vi "harp_connection_open.vi"(0 "Port:":refnum<visa-resource-name>="COMx", 1 "device's firmware name":string, 2 "launch dialog":bool, 3 ".X settings":T2={"fw .hex file path"=path "Fir", "updater path"=path "Fir"}, 7 "Expected device ID":u16=1024, 11 "MinimumVersions":T3={"hwVerMajor"=0, "fwVerMajor"=0, "harpVerMajor"=0, "assVer"=0, "hwVerMinor"=0, "fwVerMinor"=0, "harpVerMinor"=10}, 12 "get lists only":bool, 13 "baud rate":u32(ring)=1000000 items=["250Kbit/s"=250000, "500kbit/s"=500000, "1Mbit/s"=1000000, "2Mbit/s"=2000000, "4Mbit/s"=4000000]) -> (4 "port out":refnum<visa-resource-name>, 6 "Devices Name List":string[](array[string])=["Not defined", "Poke", "Multi Pwm Generator", "Wear", "12 Volts Drive", "LED Controller", "Synchronizer", "Simple Analog Generator", "Archimedes", "Clock Synchronizer", "Camera Controller", "Behavior"], 8 "cancel (T)":bool caption="Boolean", 10 "Devices WhoAmI List":u16[](array[numeric])=[0, 1024, 1040, 1056, 1072, 1088, 1104, 1121, 1136, 1152, 1168, 1216], 14 "Devices X. settings":T1(array[cluster])=[{"reg. address"=0, "address content (en)"=0, "address content (dis)"=0, "Has .X"=FALSE}, {"reg. address"=0, "address content (en)"=0, "address content (dis)"=0, "Has .X"=FALSE}, {"reg. address"=0, "address content (en)"=0, "address content (dis)"=0, "Has .X"=FALSE}, {"reg. address"=0, "address content (en)"=0, "address content (dis)"=0, "Has .X"=FALSE}, {"reg. address"=0, "address content (en)"=0, "address content (dis)"=0, "Has .X"=FALSE}, {"reg. address"=0, "address content (en)"=0, "address content (dis)"=0, "Has .X"=FALSE}, {"reg. address"=0, "address content (en)"=0, "address content (dis)"=0, "Has .X"=FALSE}, {"reg. address"=0, "address content (en)"=0, "address content (dis)"=0, "Has .X"=FALSE}, {"reg. address"=0, "address content (en)"=0, "address content (dis)"=0, "Has .X"=FALSE}, {"reg. address"=0, "address content (en)"=0, "address content (dis)"=0, "Has .X"=FALSE}, {"reg. address"=0, "address content (en)"=0, "address content (dis)"=0, "Has .X"=FALSE}, {"reg. address"=0, "address content (en)"=0, "address content (dis)"=0, "Has .X"=FALSE}, {"reg. address"=0, "address content (en)"=0, "address content (dis)"=0, "Has .X"=FALSE}, {"reg. address"=0, "address content (en)"=0, "address content (dis)"=0, "Has .X"=FALSE}, {"reg. address"=0, "address content (en)"=0, "address content (dis)"=0, "Has .X"=FALSE}, {"reg. address"=82, "address content (en)"=1, "address content (dis)"=0, "Has .X"=TRUE}, {"reg. address"=0, "address content (en)"=0, "address content (dis)"=0, "Has .X"=FALSE}], 15 "error out":errorcluster)   [LabVIEW 2010]
uses:
  <vilib>/Instr/_visa.llb/VISA Flush IO Buffer Mask.ctl
  <vilib>/Instr/_visa.llb/VISA Configure Serial Port (Instr).vi
panel:
  in  "cancel":bool caption="Boolean"
  in  "connect":bool caption="Boolean"
  # "Choose the device COM port."
  # "COM port:"
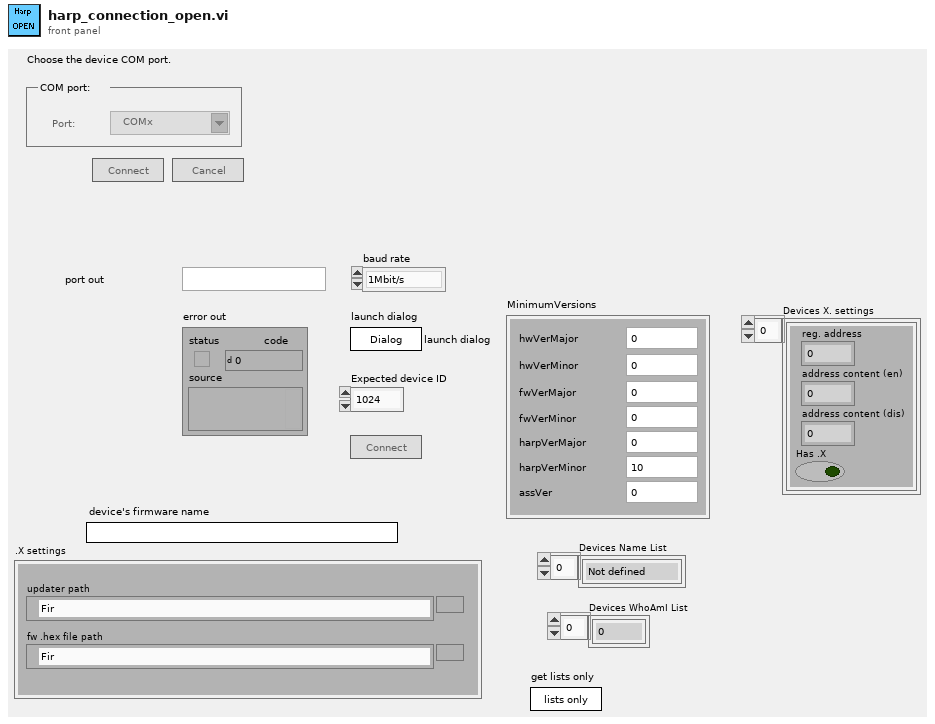
[diagram p1: front panel]
types:
  T1 = cluster{"reg. address":u8, "address content (en)":u8, "address content (dis)":u8, "Has .X":bool}[]
  T2 = cluster{"fw .hex file path":path, "updater path":path}
  T3 = cluster{"hwVerMajor":u8, "fwVerMajor":u8, "harpVerMajor":u8, "assVer":u8, "hwVerMinor":u8, "fwVerMinor":u8, "harpVerMinor":u8}
  T4 = cluster{"reg. address":u8, "address content (en)":u8, "address content (dis)":u8, "fw .hex file path":path, "updater path":path}
  T5 = enum8{"Enabled", "Disabled", "Disabled and Grayed Out"}
  T6 = typedef "VISA Flush IO Buffer Mask.ctl" = u16
  T7 = cluster{"reg. address":u8, "address content (en)":u8, "address content (dis)":u8, "Has .X":bool}
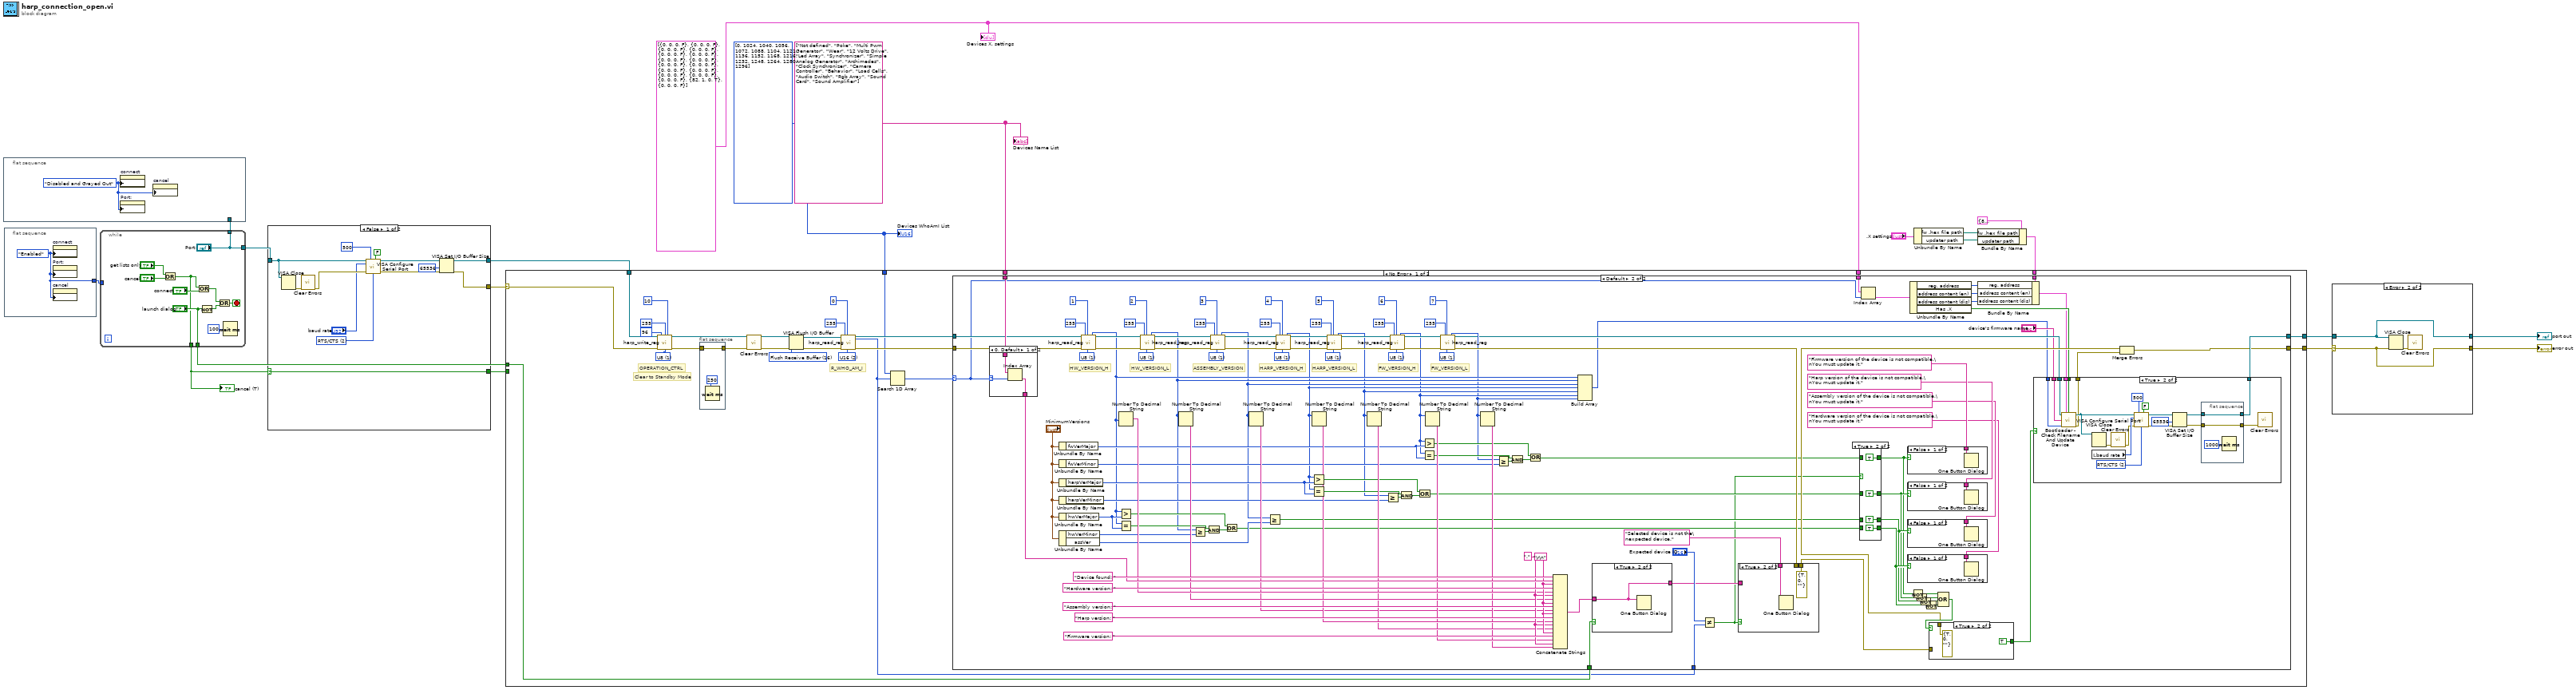
[diagram p0: block diagram]
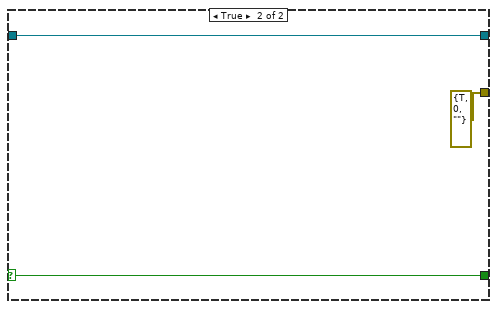
[diagram p3: hidden frame]
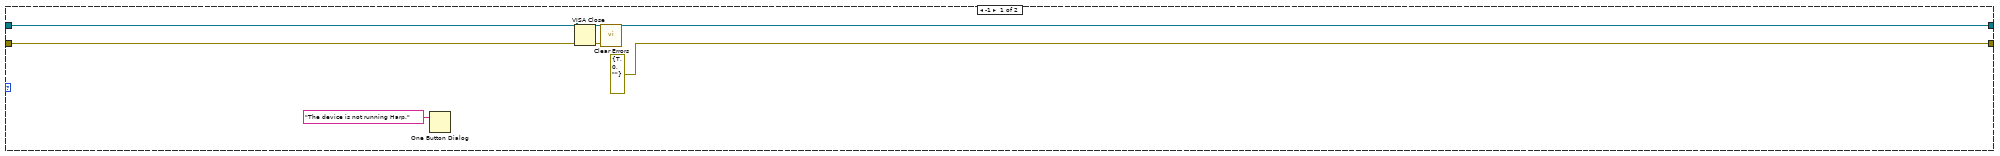
[diagram p4: hidden frame]
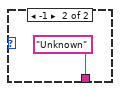
[diagram p5: hidden frame]
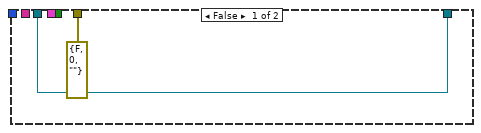
[diagram p6: hidden frame]
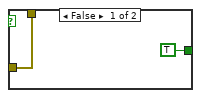
[diagram p8: hidden frame]
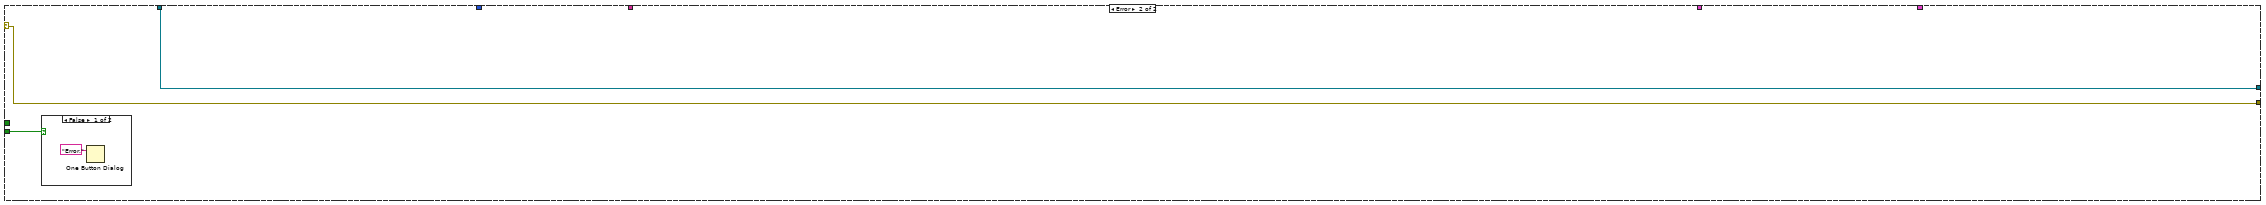
[diagram p15: hidden frame]
diagram:
  w6 = T1 [{"reg. address"=0, "address content (en)"=0, "address content (dis)"=0, "Has .X"=FALSE}, {"reg. address"=0, "address content (en)"=0, "address content (dis)"=0, "Has .X"=FALSE}, {"reg. address"=0, "address content (en)"=0, "address content (dis)"=0, "Has .X"=FALSE}, {"reg. address"=0, "address content (en)"=0, "address content (dis)"=0, "Has .X"=FALSE}, {"reg. address"=0, "address content (en)"=0, "address content (dis)"=0, "Has .X"=FALSE}, {"reg. address"=0, "address content (en)"=0, "address content (dis)"=0, "Has .X"=FALSE}, {"reg. address"=0, "address content (en)"=0, "address content (dis)"=0, "Has .X"=FALSE}, {"reg. address"=0, "address content (en)"=0, "address content (dis)"=0, "Has .X"=FALSE}, {"reg. address"=0, "address content (en)"=0, "address content (dis)"=0, "Has .X"=FALSE}, {"reg. address"=0, "address content (en)"=0, "address content (dis)"=0, "Has .X"=FALSE}, {"reg. address"=0, "address content (en)"=0, "address content (dis)"=0, "Has .X"=FALSE}, {"reg. address"=0, "address content (en)"=0, "address content (dis)"=0, "Has .X"=FALSE}, {"reg. address"=0, "address content (en)"=0, "address content (dis)"=0, "Has .X"=FALSE}, {"reg. address"=0, "address content (en)"=0, "address content (dis)"=0, "Has .X"=FALSE}, {"reg. address"=0, "address content (en)"=0, "address content (dis)"=0, "Has .X"=FALSE}, {"reg. address"=82, "address content (en)"=1, "address content (dis)"=0, "Has .X"=TRUE}, {"reg. address"=0, "address content (en)"=0, "address content (dis)"=0, "Has .X"=FALSE}] ("Array")
  w18 = string[] ["Not defined", "Poke", "Multi Pwm Generator", "Wear", "12 Volts Drive", "Led Array", "Synchronizer", "Simple Analog Generator", "Archimedes", "Clock Synchronizer", "Camera Controller", "Behavior", "Load Cells", "Audio Switch", "Rgb Array", "Sound Card", "Sound Amplifier"]
  w19 = u16[] [0, 1024, 1040, 1056, 1072, 1088, 1104, 1121, 1136, 1152, 1168, 1216, 1232, 1248, 1264, 1280, 1296]
  n1 = flat-sequence {
    tunnel: w13 -> [_]
    frame #0 {
      w21 = T5."Disabled and Grayed Out" ("Disabled")
      n2 = property on="connect" class="Bool"("DisabledEnum"=w21) -> ()  [unwired: 2 in, 2 out]
      n3 = property on="Port:" class="VISAName"("DisabledEnum"=w21) -> ()  [unwired: 2 in, 2 out]
      n4 = property on="cancel" class="Bool"("DisabledEnum"=w21) -> ()  [unwired: 2 in, 2 out]
    }
  }
  n5 = flat-sequence {
    tunnel: [w22] -> w14
    frame #0 {
      w22 = T5."Enabled" ("Disabled")
      n6 = property on="connect" class="Bool"("DisabledEnum"=w22) -> ()  [unwired: 2 in, 2 out]
      n7 = property on="Port:" class="VISAName"("DisabledEnum"=w22) -> ()  [unwired: 2 in, 2 out]
      n8 = property on="cancel" class="Bool"("DisabledEnum"=w22) -> ()  [unwired: 2 in, 2 out]
    }
  }
  n9 = while {
    tunnel: ["Port:"] -> w17
    tunnel: ["launch dialog"] -> w20
    tunnel: w14 -> [_]
    tunnel: ["Port:"] -> w13
    tunnel: [w24] -> w12
    stop <- w31 stop-if-true
    n10 = Or(x="get lists only", y="cancel") -> (x .or. y?=w24:bool)
    n11 = Or(x=w24, y="connect") -> (x .or. y?=w26:bool)
    n12 = Not(x="launch dialog") -> (.not. x?=w30:bool)
    n13 = Or(x=w26, y=w30) -> (x .or. y?=w31:bool)
    n14 = Wait (ms)(milliseconds to wait=u32 100) -> ()  [unwired: 1 out]
  }
  "cancel (T)" <- w12
  n15 = case shown="False" w12 {
    selector: w12 -> [w33 w46]
    tunnel: w17 -> [w39 w48]
    tunnel: [w36 errorcluster {"status"=TRUE, "code"=0, "source"=""} ("error out")] -> w16
    tunnel: [w35 w48] -> w15
    tunnel: [w33 w46] -> w11
    frame False {
      w41 = u16 2 items=["None", "XON/XOFF", "RTS/CTS", "XON/XOFF & RTS/CTS", "DTR/DSR", "XON/XOFF & DTR/DSR"] ("flow control (0:none)")
      n16 = VISA Close(VISA resource name=w39) -> (error out=w42:errorcluster)  [unwired: 1 in]
      n17 = call <vilib>:"Clear Errors.vi"("error in (no error)"=w42) -> ("error out"=w44:errorcluster)  [unwired: 6 in]
      n18 = call-poly "VISA Configure Serial Port"("VISA resource name"=w39, "timeout (10sec)"=u32 500, "Enable Termination\nChar (T)"=FALSE ("Enable Termination\nChar (T)"), "baud rate (9600)"="baud rate", "error in (no error)"=w44, "flow control (0:none)"=w41) -> ("VISA resource name out"=w37:refnum<visa-resource-name>, "error out"=w38:errorcluster)  [unwired: 8 in]
      n19 = VISA Set I/O Buffer Size(VISA resource name=w37, size (4096)=u32 65536, error in (no error)=w38) -> (VISA resource name out=w35:refnum<visa-resource-name>, error out=w36:errorcluster)  [unwired: 1 in]
    }
    frame True {
    }
  }
  n20 = Unbundle By Name(".X settings") -> ("fw .hex file path"=w3:path, "updater path"=w4:path)
  n21 = Bundle By Name(cluster=T4 {"reg. address"=82, "address content (en)"=1, "address content (dis)"=0, "fw .hex file path"=path "C:/Users/Filipe Carvalho/Desktop/Bitbucket.Soundcard/Firmware.PIC32/firmware/SoundCard.X/dist/default/production/SoundCard.X.production.hex", "updater path"=path "C:/Users/Filipe Carvalho/Documents/HarpSoundCard/Updater"} (".X settings 2"), "fw .hex file path"=w3, "updater path"=w4) -> (w1:T4)
  n22 = case shown="No Error" w16 {
    selector: w16 -> [w53 w256]
    tunnel: w20 -> [w68 _]
    tunnel: w15 -> [w54 w255]
    tunnel: w19 -> [w70 _]
    tunnel: w18 -> [w69 _]
    tunnel: [w66 w256] -> w9
    tunnel: [w65 w255] -> w10
    tunnel: w11 -> [_ w254]
    tunnel: w6 -> [w50 _]
    tunnel: w1 -> [w49 _]
    frame No Error {
      w58 = T6 16 items=["Flush Receive Buffer"=16, "Write Transmit Buffer to Device"=32, "Flush Receive Buffer (No I/O)"=64, "Flush Transmit Buffer"=128] ("Mask")
      w62 = u8 1 items=["U8"=1, "U16"=2, "U32"=4, "U64"=8, "I8"=129, "I16"=130, "I32"=132, "I64"=136, "FLOAT"=68, "BOOL"=17] ("type")
      w75 = u8 2 items=["U8"=1, "U16"=2, "U32"=4, "U64"=8, "I8"=129, "I16"=130, "I32"=132, "I64"=136, "FLOAT"=68, "BOOL"=17] ("type")
      # "Clear to Standby Mode"
      # "OPERATION_CTRL"
      # "R_WHO_AM_I"
      n23 = call "harp_write_reg.vi"(0:"port"=w54, "error in (no error)"=w53, "8 bits"=u8 96 ("y"), 10:"port"=u8 255 ("port"), "type"=w62, "reg. address"=u8 10) -> ("port out"=w63:refnum<visa-resource-name>, "error out"=w64:errorcluster)  [unwired: 11 in, 1 out]
      n24 = flat-sequence {
        tunnel: [w76] -> w59
        tunnel: w64 -> [w76]
        frame #0 {
          n25 = Wait (ms)(milliseconds to wait=u32 250) -> ()  [unwired: 1 out]
        }
      }
      n26 = call <vilib>:"Clear Errors.vi"("error in (no error)"=w59) -> ("error out"=w52:errorcluster)  [unwired: 6 in]
      n27 = VISA Flush I/O Buffer(VISA resource name=w63, mask (16)=w58, error in (no error)=w52) -> (VISA resource name out=w55:refnum<visa-resource-name>, error out=w56:errorcluster)
      n28 = call "harp_read_reg.vi"(0:"port"=w55, "error in (no error)"=w56, 6:"port"=u8 255 ("port"), "reg. address"=u8 0, "type"=w75) -> ("port out"=w72:refnum<visa-resource-name>, "16 bits"=w67:u16, "error out"=w71:errorcluster)  [unwired: 5 in, 7 out]
      n29 = Search 1D Array(1D array=w70, element=w67) -> (index of element=w51:i32)  [unwired: 1 in]
      n30 = case shown="Default" w51 {
        selector: w51 -> [_ w91]
        tunnel: w72 -> [w81 w154]
        tunnel: w71 -> [w80 w155]
        tunnel: w69 -> [_ w186]
        tunnel: w68 -> [_ w183]
        tunnel: w67 -> [_ w181]
        tunnel: [errorcluster {"status"=TRUE, "code"=0, "source"=""} ("error out") w93] -> w66
        tunnel: [w81 w94] -> w65
        tunnel: w50 -> [_ w90]
        tunnel: w49 -> [_ w85]
        frame -1 {
          n31 = One Button Dialog(message="The device is not running Harp.") -> ()  [unwired: 1 in, 1 out]
          n32 = VISA Close(VISA resource name=w81, error in (no error)=w80) -> (error out=w78:errorcluster)
          n33 = call <vilib>:"Clear Errors.vi"("error in (no error)"=w78) -> ()  [unwired: 6 in, 1 out]
        }
        frame Default {
          w166 = u8 1 items=["U8"=1, "U16"=2, "U32"=4, "U64"=8, "I8"=129, "I16"=130, "I32"=132, "I64"=136, "FLOAT"=68, "BOOL"=17] ("type")
          w174 = u8 1 items=["U8"=1, "U16"=2, "U32"=4, "U64"=8, "I8"=129, "I16"=130, "I32"=132, "I64"=136, "FLOAT"=68, "BOOL"=17] ("type")
          w175 = u8 1 items=["U8"=1, "U16"=2, "U32"=4, "U64"=8, "I8"=129, "I16"=130, "I32"=132, "I64"=136, "FLOAT"=68, "BOOL"=17] ("type")
          w156 = "."
          w158 = "\r\n"
          w193 = u8 1 items=["U8"=1, "U16"=2, "U32"=4, "U64"=8, "I8"=129, "I16"=130, "I32"=132, "I64"=136, "FLOAT"=68, "BOOL"=17] ("type")
          w192 = u8 1 items=["U8"=1, "U16"=2, "U32"=4, "U64"=8, "I8"=129, "I16"=130, "I32"=132, "I64"=136, "FLOAT"=68, "BOOL"=17] ("type")
          w200 = u8 1 items=["U8"=1, "U16"=2, "U32"=4, "U64"=8, "I8"=129, "I16"=130, "I32"=132, "I64"=136, "FLOAT"=68, "BOOL"=17] ("type")
          w201 = u8 1 items=["U8"=1, "U16"=2, "U32"=4, "U64"=8, "I8"=129, "I16"=130, "I32"=132, "I64"=136, "FLOAT"=68, "BOOL"=17] ("type")
          # "HW_VERSION_L"
          # "FW_VERSION_L"
          # "FW_VERSION_H"
          # "HARP_VERSION_L"
          # "HARP_VERSION_H"
          # "ASSEMBLY_VERSION"
          # "HW_VERSION_H"
          n34 = case shown="0, Default" w91 {
            selector: w91 -> [w204 _]
            tunnel: w186 -> [w206 _]
            tunnel: [w205 "Unknown" ("message")] -> w184
            frame 0, Default {
              n35 = Index Array(array=w206, index=w204) -> (element=w205:string)
            }
            frame -1 {
            }
          }
          n36 = Unbundle By Name("MinimumVersions") -> ("fwVerMajor"=w125:u8)
          n37 = Unbundle By Name("MinimumVersions") -> ("fwVerMinor"=w124:u8)
          n38 = Unbundle By Name("MinimumVersions") -> ("harpVerMajor"=w126:u8)
          n39 = Unbundle By Name("MinimumVersions") -> ("harpVerMinor"=w127:u8)
          n40 = Unbundle By Name("MinimumVersions") -> ("hwVerMajor"=w138:u8)
          n41 = Unbundle By Name("MinimumVersions") -> ("hwVerMinor"=w137:u8, "assVer"=w132:u8)
          n42 = call "harp_read_reg.vi"(0:"port"=w154, "error in (no error)"=w155, 6:"port"=u8 255 ("port"), "reg. address"=u8 1, "type"=w201) -> ("8 bits"=w105:u8, "port out"=w164:refnum<visa-resource-name>, "error out"=w165:errorcluster)  [unwired: 5 in, 7 out]
          n43 = Number To Decimal String(number=w105) -> (decimal integer string=w153:string)  [unwired: 1 in]
          n44 = Greater?(x=w105, y=w138) -> (0:w133:bool)
          n45 = Equal?(x=w105, y=w138) -> (x = y?=w136:bool)
          n46 = call "harp_read_reg.vi"(0:"port"=w164, "error in (no error)"=w165, 6:"port"=u8 255 ("port"), "reg. address"=u8 2, "type"=w166) -> ("8 bits"=w104:u8, "port out"=w163:refnum<visa-resource-name>, "error out"=w162:errorcluster)  [unwired: 5 in, 7 out]
          n47 = Number To Decimal String(number=w104) -> (decimal integer string=w152:string)  [unwired: 1 in]
          n48 = Greater Or Equal?(x=w104, y=w137) -> (x >= y?=w135:bool)
          n49 = And(x=w136, y=w135) -> (x .and. y?=w134:bool)
          n50 = call "harp_read_reg.vi"(0:"port"=w163, "error in (no error)"=w162, 6:"port"=u8 255 ("port"), "reg. address"=u8 3, "type"=w200) -> ("8 bits"=w103:u8, "port out"=w188:refnum<visa-resource-name>, "error out"=w189:errorcluster)  [unwired: 5 in, 7 out]
          n51 = Or(x=w133, y=w134) -> (x .or. y?=w114:bool)
          n52 = Number To Decimal String(number=w103) -> (decimal integer string=w147:string)  [unwired: 1 in]
          n53 = Greater Or Equal?(x=w103, y=w132) -> (x >= y?=w113:bool)
          n54 = call "harp_read_reg.vi"(0:"port"=w188, "error in (no error)"=w189, 6:"port"=u8 255 ("port"), "reg. address"=u8 4, "type"=w192) -> ("8 bits"=w102:u8, "port out"=w196:refnum<visa-resource-name>, "error out"=w197:errorcluster)  [unwired: 5 in, 7 out]
          n55 = Number To Decimal String(number=w102) -> (decimal integer string=w151:string)  [unwired: 1 in]
          n56 = Greater?(x=w102, y=w126) -> (0:w131:bool)
          n57 = Equal?(x=w102, y=w126) -> (x = y?=w128:bool)
          n58 = call "harp_read_reg.vi"(0:"port"=w196, "error in (no error)"=w197, 6:"port"=u8 255 ("port"), "reg. address"=u8 5, "type"=w193) -> ("8 bits"=w101:u8, "port out"=w168:refnum<visa-resource-name>, "error out"=w169:errorcluster)  [unwired: 5 in, 7 out]
          n59 = Number To Decimal String(number=w101) -> (decimal integer string=w150:string)  [unwired: 1 in]
          n60 = Greater Or Equal?(x=w101, y=w127) -> (x >= y?=w129:bool)
          n61 = call "harp_read_reg.vi"(0:"port"=w168, "error in (no error)"=w169, 6:"port"=u8 255 ("port"), "reg. address"=u8 6, "type"=w175) -> ("8 bits"=w100:u8, "port out"=w171:refnum<visa-resource-name>, "error out"=w170:errorcluster)  [unwired: 5 in, 7 out]
          n62 = And(x=w128, y=w129) -> (x .and. y?=w130:bool)
          n63 = Or(x=w131, y=w130) -> (x .or. y?=w112:bool)
          n64 = Greater?(x=w100, y=w125) -> (0:w120:bool)
          n65 = Equal?(x=w100, y=w125) -> (x = y?=w123:bool)
          n66 = Number To Decimal String(number=w100) -> (decimal integer string=w149:string)  [unwired: 1 in]
          n67 = call "harp_read_reg.vi"(0:"port"=w171, "error in (no error)"=w170, 6:"port"=u8 255 ("port"), "reg. address"=u8 7, "type"=w174) -> ("8 bits"=w99:u8, "port out"=w98:refnum<visa-resource-name>, "error out"=w146:errorcluster)  [unwired: 5 in, 7 out]
          n68 = Number To Decimal String(number=w99) -> (decimal integer string=w148:string)  [unwired: 1 in]
          n69 = Greater Or Equal?(x=w99, y=w124) -> (x >= y?=w122:bool)
          n70 = And(x=w123, y=w122) -> (x .and. y?=w121:bool)
          n71 = Or(x=w120, y=w121) -> (x .or. y?=w111:bool)
          n72 = Concatenate Strings("Device found: " ("string"), w184, w158, "Hardware version: " ("string"), w153, w156, w152, w158, "Assembly version: " ("string"), w147, w158, "Harp version: " ("string"), w151, w156, w150, w158, "Firmware version: " ("string"), w149, w156, w148) -> (w182:string)
          n73 = Build Array(w105, w104, w103, w102, w101, w100, w99) -> (w95:u8[])
          n74 = case shown="True" w183 {
            tunnel: w182 -> [w252 w253]
            tunnel: [w252 w253] -> w178
            frame False {
            }
            frame True {
              n75 = One Button Dialog(message=w253) -> ()  [unwired: 1 in, 1 out]
            }
          }
          n76 = Not Equal?(x="Expected device ID", y=w181) -> (x != y?=w106:bool)
          n77 = case shown="True" w106 {
            tunnel: "Selected device is not the\nexpected device." -> [_ w251]
            tunnel: w178 -> [_ _]
            tunnel: [w249 errorcluster {"status"=TRUE, "code"=0, "source"=""} ("error out")] -> w140
            tunnel: w146 -> [w249 _]
            frame False {
            }
            frame True {
              n78 = One Button Dialog(message=w251) -> ()  [unwired: 1 in, 1 out]
            }
          }
          n79 = case shown="True" w106 {
            tunnel: w114 -> [w236 _]
            tunnel: w113 -> [w235 _]
            tunnel: w112 -> [w234 _]
            tunnel: w111 -> [w233 _]
            tunnel: [w236 TRUE] -> w110
            tunnel: [w235 TRUE] -> w109
            tunnel: [w234 TRUE] -> w108
            tunnel: [w233 TRUE] -> w107
            frame False {
            }
            frame True {
            }
          }
          n80 = Index Array(array=w90, index=w91) -> (element=w89:T7)
          n81 = case shown="False" w107 {
            tunnel: "Firmware version of the device is not compatible.\nYou must update it." -> [w248 _]
            frame False {
              n82 = One Button Dialog(message=w248) -> ()  [unwired: 1 in, 1 out]
            }
            frame True {
            }
          }
          n83 = case shown="False" w108 {
            tunnel: "Harp version of the device is not compatible.\nYou must update it." -> [w247 _]
            frame False {
              n84 = One Button Dialog(message=w247) -> ()  [unwired: 1 in, 1 out]
            }
            frame True {
            }
          }
          n85 = case shown="False" w109 {
            tunnel: "Assembly version of the device is not compatible.\nYou must update it." -> [w246 _]
            frame False {
              n86 = One Button Dialog(message=w246) -> ()  [unwired: 1 in, 1 out]
            }
            frame True {
            }
          }
          n87 = case shown="False" w110 {
            tunnel: "Hardware version of the device is not compatible.\nYou must update it." -> [w245 _]
            frame False {
              n88 = One Button Dialog(message=w245) -> ()  [unwired: 1 in, 1 out]
            }
            frame True {
            }
          }
          n89 = Unbundle By Name(w89) -> ("reg. address"=w86:u8, "address content (en)"=w87:u8, "address content (dis)"=w88:u8, "Has .X"=w84:bool)
          n90 = Not(x=w107) -> (.not. x?=w118:bool)
          n91 = Not(x=w108) -> (.not. x?=w117:bool)
          n92 = Not(x=w109) -> (.not. x?=w116:bool)
          n93 = Not(x=w110) -> (.not. x?=w115:bool)
          n94 = Compound Arithmetic op=OR(w118, w117, w116, w115) -> (w141:bool)
          n95 = case shown="True" w141 {
            tunnel: [w242 errorcluster {"status"=TRUE, "code"=0, "source"=""} ("error out")] -> w139
            tunnel: w140 -> [w242 _]
            tunnel: [TRUE TRUE] -> w97
            frame False {
            }
            frame True {
            }
          }
          n96 = Bundle By Name(cluster=w85, "reg. address"=w86, "address content (en)"=w87, "address content (dis)"=w88) -> (w83:T4)
          n97 = case shown="True" w97 {
            tunnel: w98 -> [w209 w219]
            tunnel: "device's firmware name" -> [_ w218]
            tunnel: w95 -> [_ w217]
            tunnel: [w209 w216] -> w94
            tunnel: [errorcluster {"status"=FALSE, "code"=0, "source"=""} ("error out") w212] -> w92
            tunnel: w84 -> [_ w211]
            tunnel: w83 -> [_ w210]
            frame False {
            }
            frame True {
              w224 = u16 2 items=["None", "XON/XOFF", "RTS/CTS", "XON/XOFF & RTS/CTS", "DTR/DSR", "XON/XOFF & DTR/DSR"] ("flow control (0:none)")
              n98 = call "Bootloader - Check Filename And Update Device.vi"("VISA resource name"=w219, ".X settings"=w210, "Device has .X"=w211, "device name"=w218, "current versions"=w217) -> ("VISA resource name"=w220:refnum<visa-resource-name>, "error out"=w212:errorcluster)  [unwired: 9 in]
              n99 = VISA Close(VISA resource name=w220) -> (error out=w225:errorcluster)  [unwired: 1 in]
              n100 = local read "baud rate"() -> (w229:u32)
              n101 = call <vilib>:"Clear Errors.vi"("error in (no error)"=w225) -> ("error out"=w227:errorcluster)  [unwired: 6 in]
              n102 = call-poly "VISA Configure Serial Port"("VISA resource name"=w220, "timeout (10sec)"=u32 500, "Enable Termination\nChar (T)"=FALSE ("Enable Termination\nChar (T)"), "baud rate (9600)"=w229, "error in (no error)"=w227, "flow control (0:none)"=w224) -> ("VISA resource name out"=w222:refnum<visa-resource-name>, "error out"=w223:errorcluster)  [unwired: 8 in]
              n103 = VISA Set I/O Buffer Size(VISA resource name=w222, size (4096)=u32 65536, error in (no error)=w223) -> (VISA resource name out=w215:refnum<visa-resource-name>, error out=w213:errorcluster)  [unwired: 1 in]
              n104 = flat-sequence {
                tunnel: [w231] -> w216
                tunnel: w215 -> [w231]
                tunnel: [w230] -> w214
                tunnel: w213 -> [w230]
                frame #0 {
                  n105 = Wait (ms)(milliseconds to wait=u32 1000) -> ()  [unwired: 1 out]
                }
              }
              n106 = call <vilib>:"Clear Errors.vi"("error in (no error)"=w214) -> ()  [unwired: 6 in, 1 out]
            }
          }
          n107 = Merge Errors(w139, w92) -> (w93:errorcluster)
        }
      }
    }
    frame Error {
      n108 = case shown="False" w254 {
        frame False {
          n109 = One Button Dialog(message="Error.") -> ()  [unwired: 1 in, 1 out]
        }
        frame True {
        }
      }
    }
  }
  n110 = case shown="Error" w9 {
    selector: w9 -> [w259 w261]
    tunnel: w10 -> [w258 w260]
    tunnel: [w259 w261] -> w8
    tunnel: [w258 w260] -> w7
    frame No Error {
    }
    frame Error {
      n111 = VISA Close(VISA resource name=w260, error in (no error)=w261) -> (error out=w262:errorcluster)
      n112 = call <vilib>:"Clear Errors.vi"("error in (no error)"=w262) -> ()  [unwired: 6 in, 1 out]
    }
  }
  "port out" <- w7
  "error out" <- w8
  "Devices Name List" <- w18
  "Devices WhoAmI List" <- w19
  "Devices X. settings" <- w6
